vi "Read List Points.vi"(8 "error in (no error)":errorcluster, 9 "List (0: Current List)":i32(ring) items=["Current List", "Dwell List", "Voltage List", "Begin Step Trigger List", "End Step Trigger List"], 10 "Channel (1)":string="1", 11 "VISA resource name":refnum<visa-resource-name>) -> (0 "error out":errorcluster, 2 "Points Number":i32[](array[numeric]), 3 "VISA resource name out":refnum<visa-resource-name>)   [LabVIEW 2020, in "Keysight E36300 Series.lvlib"]
doc: "Returns the number of points (steps) in the specified list, not the point values.\n\n<b>Note: </b>\nThis VI is only applicable for E36312A and E36313A models."
uses:
  Keysight E36300 Series.lvlib
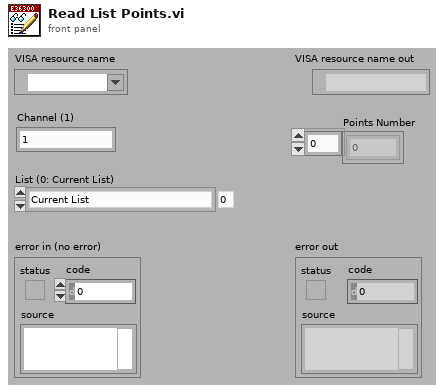
[diagram p1: front panel]
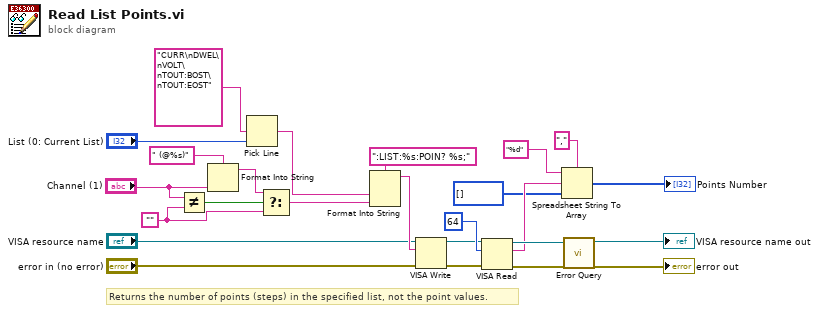
[diagram p0: block diagram]
diagram:
  w2 = ""
  # "Returns the number of points (steps) in the specified list, not the point values."
  n1 = Not Equal?(x="Channel (1)", y=w2) -> (x != y?=w4:bool)
  n2 = Format Into String(format string=" (@%s)", "Channel (1)") -> (resulting string=w5:string)  [unwired: 2 in, 1 out]
  n3 = Pick Line(multi-line string="CURR\nDWEL\nVOLT\nTOUT:BOST\nTOUT:EOST", line index="List (0: Current List)") -> (output string=w22:string)  [unwired: 1 in]
  n4 = Select(t=w5, s=w4, f=w2) -> (s? t:f=w1:string)
  n5 = Format Into String(format string=":LIST:%s:POIN? %s;", w22, w1) -> (resulting string=w21:string)  [unwired: 2 in, 1 out]
  n6 = VISA Write(VISA resource name="VISA resource name", write buffer=w21, error in (no error)="error in (no error)") -> (VISA resource name out=w15:refnum<visa-resource-name>, error out=w14:errorcluster)  [unwired: 1 out]
  n7 = VISA Read(VISA resource name=w15, byte count=u32 64, error in (no error)=w14) -> (VISA resource name out=w12:refnum<visa-resource-name>, read buffer=w9:string, error out=w13:errorcluster)  [unwired: 1 out]
  n8 = Spreadsheet String To Array(delimiter (Tab)=",", format string="%d", spreadsheet string=w9, array type (2D Dbl)=i32[] []) -> (array=→"Points Number":i32[])
  n9 = call "Error Query.vi"("error in (no error)"=w13, "VISA resource name"=w12) -> ("error out"=→"error out":errorcluster, "VISA resource name out"=→"VISA resource name out":refnum<visa-resource-name>)  [unwired: 6 in, 2 out]
